vi "GetData.vi"(8 "File":path=path "10 Ft", 11 "file (use dialog)":path) -> (0 "Acceleration Limit (fps^2)":dbl, 1 "Sample Period (s)":dbl, 2 "Velocity Limit (fps)":dbl, 3 "Trajectory Data":T4(array[cluster]), 4 "Commands":cluster{"Time (s)":dbl, T2, bool}[](array[cluster]), 5 "Points":cluster{"x":dbl, "y":dbl, "th":dbl}[](array[cluster]), 6 "Description":string, 7 "Cluster":cluster{"Time (s)":dbl, "Distance (ft)":dbl}, 9 "Cluster 2":T1)   [LabVIEW 2019]
doc: "Getting trajectory data from the roboRio"
uses:
  Bordeaux/Command Stuff/Single Cmd Info.ctl
  <vilib>/picture/picture.llb/imagedata.ctl
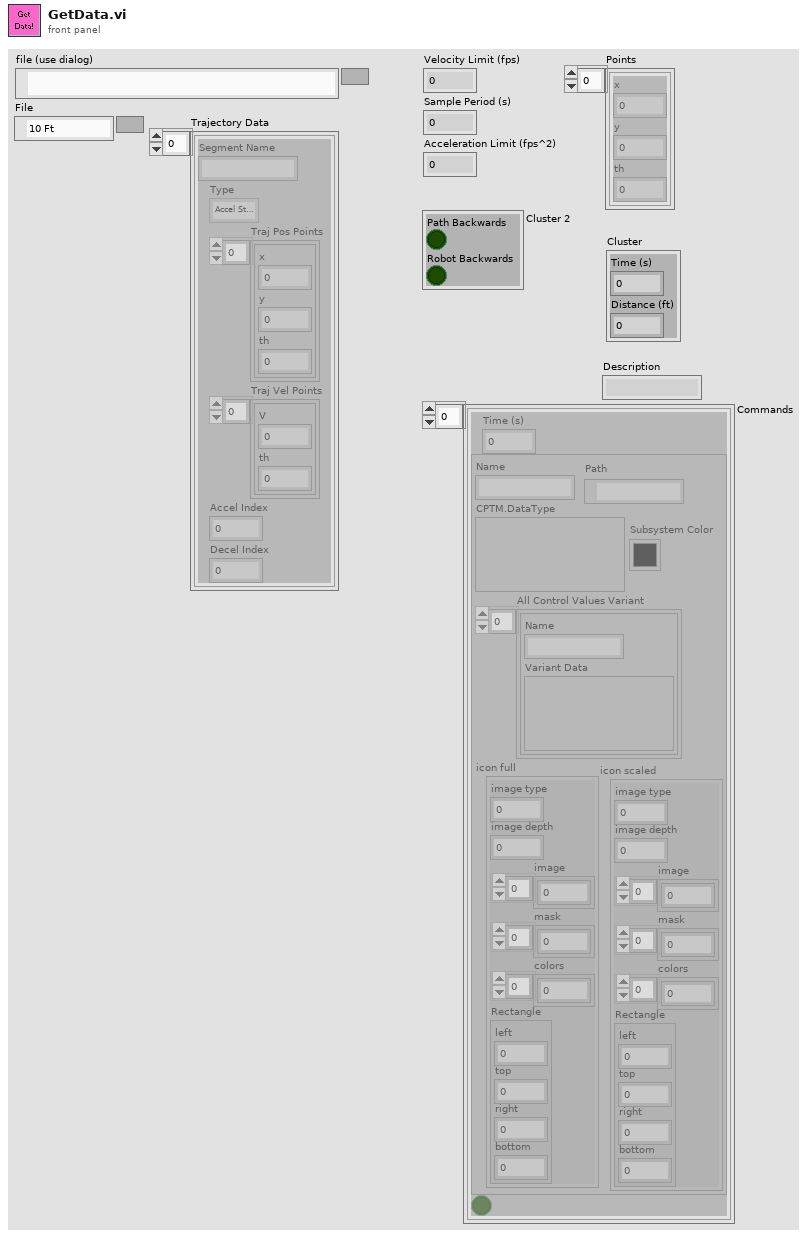
[diagram p1: front panel]
types:
  T1 = cluster{"Path Backwards":bool, "Robot Backwards":bool}
  T2 = typedef "Single Cmd Info.ctl" = cluster{"Name":string, "CPTM.DataType":variant, "All Control Values Variant":cluster{"Name":string, "Variant Data":variant}[], "icon full":T3, "icon scaled":T3, "Path":path, "Subsystem Color":u32}
  T3 = typedef "imagedata.ctl" = cluster{"image type":i32, "image depth":i32, "image":u8[], "mask":u8[], "colors":u32[], "Rectangle":cluster{"left":i16, "top":i16, "right":i16, "bottom":i16}}
  T4 = cluster{"Segment Name":string, "Type":enum16{"Accel Straight", "Const Straight", "Blend", "Circle"}, "Traj Pos Points":cluster{"x":dbl, "y":dbl, "th":dbl}[], "Traj Vel Points":cluster{"V":dbl, "th":dbl}[], "Accel Index":i32, "Decel Index":i32}[]
  T5 = cluster{"Sample Period (s)":dbl, "Limits":cluster{"Velocity (fps)":dbl, "Acceleration (fps^2)":dbl, "Jerk (fps^3)":dbl}, "Conditions":cluster{"vInitial (fps)":dbl, "vFinal (fps)":dbl}}
  T6 = cluster{"Velocity Limit (fps)":dbl, "Sample Period (s)":dbl, "Acceleration Limit (fps^2)":dbl}
  T7 = cluster{"Sample Period (s)":dbl, "Limits":cluster{"Velocity (fps)":dbl, "Acceleration (fps^2)":dbl, "Jerk (fps^3)":dbl}, "Conditions":cluster{"vInitial (fps)":dbl, "vFinal (fps)":dbl}, "Min Rads":dbl[]}
  T8 = cluster{"Sample Period (s)":dbl, "Limits":cluster{"Velocity (fps)":dbl, "Acceleration (fps^2)":dbl, "Jerk (fps^3)":dbl}, "Conditions":cluster{"vInitial (fps)":dbl, "vFinal (fps)":dbl}, "Angular Accelerations":cluster{"Angular \nAccelerations":dbl[], "Override Limits?":bool[]}}
  T9 = cluster{"Time into Path":dbl, "System":u16, "Item Selected?":bool, "System Selection":u16}[]
  T10 = cluster{"Velocity (fps)":dbl, "Acceleration (fps^2)":dbl, "Jerk (fps^3)":dbl}
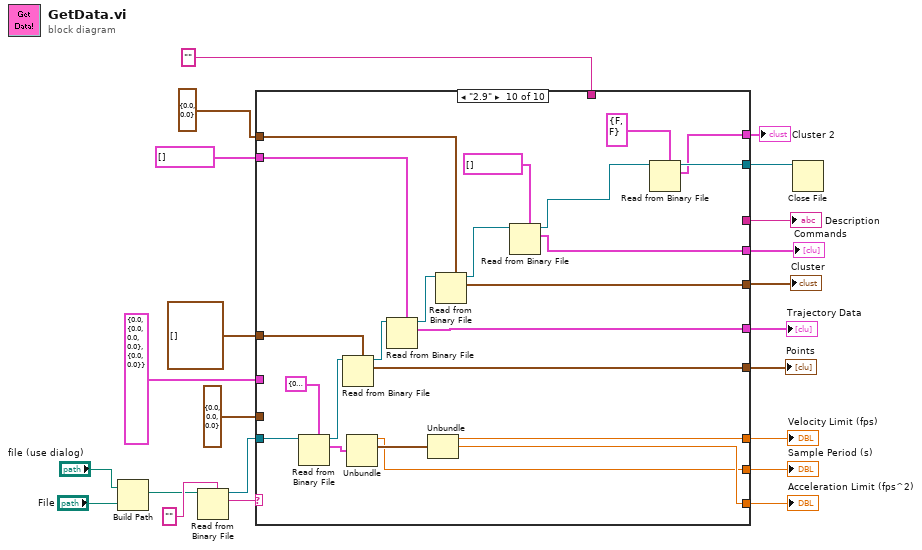
[diagram p0: block diagram]
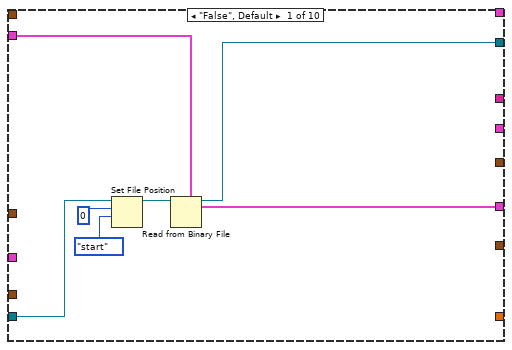
[diagram p2: hidden frame]
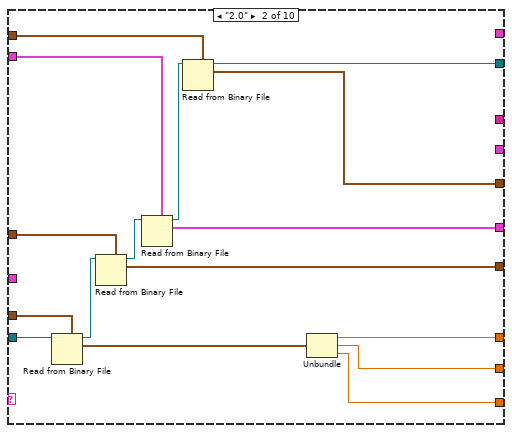
[diagram p3: hidden frame]
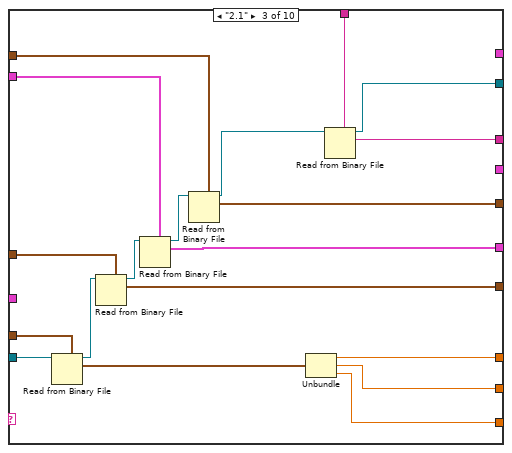
[diagram p4: hidden frame]
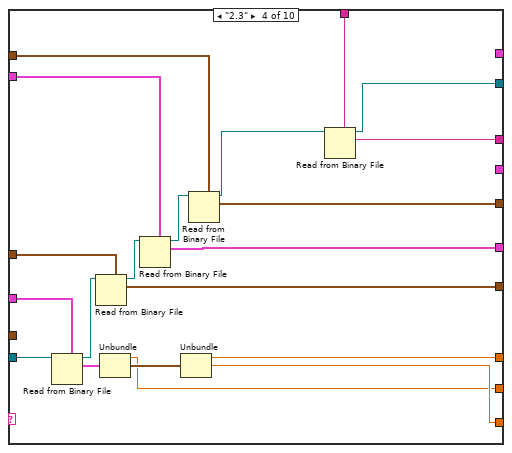
[diagram p5: hidden frame]
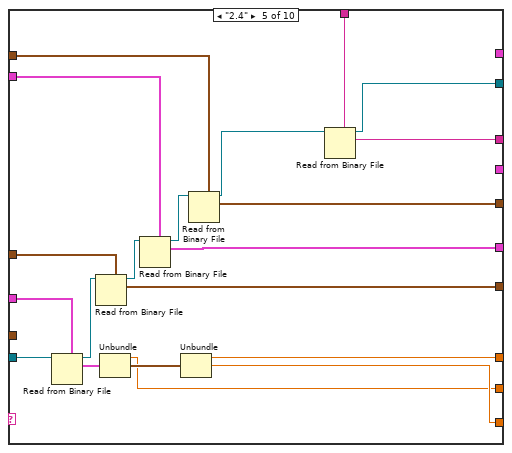
[diagram p6: hidden frame]
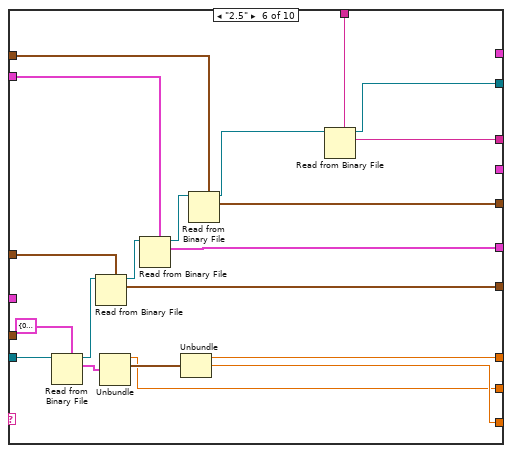
[diagram p7: hidden frame]
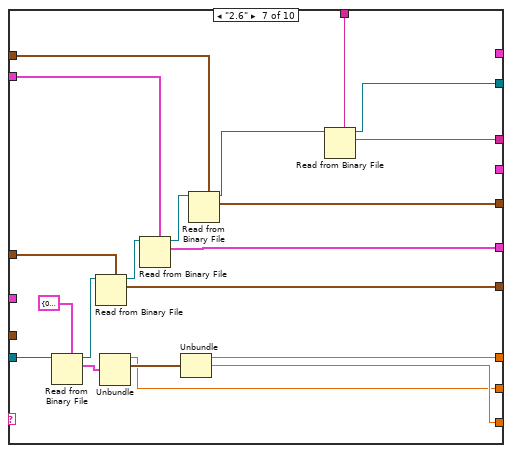
[diagram p8: hidden frame]
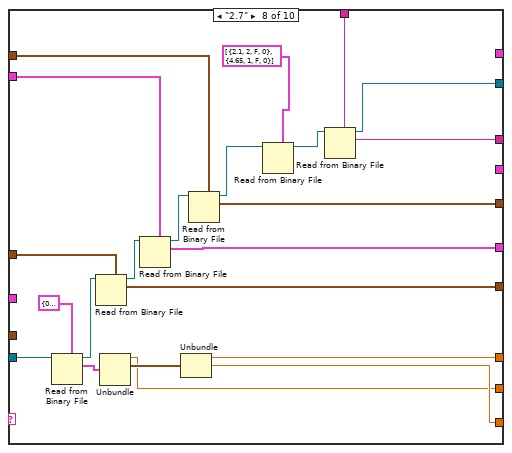
[diagram p9: hidden frame]
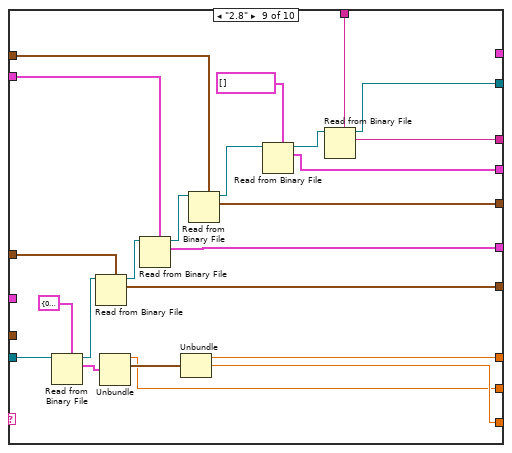
[diagram p10: hidden frame]
diagram:
  n1 = Build Path(base path="file (use dialog)", name or relative path="File") -> (appended path=w5:path)
  n2 = Read from Binary File(5:"", 11:w5) -> (2:w21:string, 3:w20:refnum<file>)  [unwired: 4 in, 2 out]
  n3 = case shown="\"2.9\"" w21 {
    tunnel: w20 -> [w24 w44 w63 w83 w103 w123 w143 w165 w188 w211]
    tunnel: T6 {"Velocity Limit (fps)"=0.0, "Sample Period (s)"=0.0, "Acceleration Limit (fps^2)"=0.0} -> [_ w43 w62 _ _ _ _ _ _ _]
    tunnel: cluster{"x":dbl, "y":dbl, "th":dbl}[] [] ("Points") -> [_ w41 w60 w81 w101 w121 w141 w163 w186 w209]
    tunnel: [_ w40 w59 w80 w100 w120 w140 w162 w185 w208] -> w11
    tunnel: T4 [] ("Trajectory Data") -> [w26 w39 w58 w79 w99 w119 w139 w161 w184 w207]
    tunnel: [w25 w37 w56 w77 w97 w117 w137 w159 w182 w205] -> w10
    tunnel: cluster{"Time (s)":dbl, "Distance (ft)":dbl} {"Time (s)"=0.0, "Distance (ft)"=0.0} -> [_ w36 w55 w76 w96 w116 w136 w158 w181 w204]
    tunnel: [_ w34 w53 w74 w94 w114 w134 w156 w179 w202] -> w9
    tunnel: [w23 w33 w48 w72 w92 w112 w132 w155 w178 w193] -> w18
    tunnel: [_ w32 w52 w67 w87 w108 w128 w151 w174 w200] -> w14
    tunnel: [_ w31 w51 w65 w85 w106 w126 w149 w172 w198] -> w13
    tunnel: [_ w30 w50 w66 w86 w107 w127 w150 w173 w199] -> w12
    tunnel: "" -> [_ _ w47 w71 w91 w111 w131 w154 w177 _]
    tunnel: [_ _ w46 w70 w90 w110 w130 w153 w176 _] -> w7
    tunnel: T5 {"Sample Period (s)"=0.0, "Limits"={"Velocity (fps)"=0.0, "Acceleration (fps^2)"=0.0, "Jerk (fps^3)"=0.0}, "Conditions"={"vInitial (fps)"=0.0, "vFinal (fps)"=0.0}} -> [_ _ _ w69 w89 _ _ _ _ _]
    tunnel: [_ _ _ _ _ _ _ _ w167 w194] -> w2
    tunnel: [_ _ _ _ _ _ _ _ _ w191] -> w1
    frame "False", Default {
      n4 = Set File Position(offset (in bytes) (0)=i64 0, refnum=w24, from (0:start)=enum16{"start", "end", "current"}."start") -> (refnum out=w27:refnum<file>)  [unwired: 1 in, 1 out]
      n5 = Read from Binary File(5:w26, 11:w27) -> (2:w25:T4, 3:w23:refnum<file>)  [unwired: 4 in, 2 out]
    }
    frame "2.0" {
      n6 = Read from Binary File(5:w43, 11:w44) -> (2:w45:T6, 3:w42:refnum<file>)  [unwired: 4 in, 2 out]
      n7 = Read from Binary File(5:w41, 11:w42) -> (2:w40:cluster{"x":dbl, "y":dbl, "th":dbl}[], 3:w38:refnum<file>)  [unwired: 4 in, 2 out]
      n8 = Read from Binary File(5:w39, 11:w38) -> (2:w37:T4, 3:w35:refnum<file>)  [unwired: 4 in, 2 out]
      n9 = Read from Binary File(5:w36, 11:w35) -> (2:w34:cluster{"Time (s)":dbl, "Distance (ft)":dbl}, 3:w33:refnum<file>)  [unwired: 4 in, 2 out]
      n10 = Unbundle(w45) -> ("Velocity Limit (fps)"=w32:dbl, "Sample Period (s)"=w31:dbl, "Acceleration Limit (fps^2)"=w30:dbl)
    }
    frame "2.1" {
      n11 = Read from Binary File(5:w62, 11:w63) -> (2:w64:T6, 3:w61:refnum<file>)  [unwired: 4 in, 2 out]
      n12 = Read from Binary File(5:w60, 11:w61) -> (2:w59:cluster{"x":dbl, "y":dbl, "th":dbl}[], 3:w57:refnum<file>)  [unwired: 4 in, 2 out]
      n13 = Read from Binary File(5:w58, 11:w57) -> (2:w56:T4, 3:w54:refnum<file>)  [unwired: 4 in, 2 out]
      n14 = Read from Binary File(5:w55, 11:w54) -> (2:w53:cluster{"Time (s)":dbl, "Distance (ft)":dbl}, 3:w49:refnum<file>)  [unwired: 4 in, 2 out]
      n15 = Unbundle(w64) -> ("Velocity Limit (fps)"=w52:dbl, "Sample Period (s)"=w51:dbl, "Acceleration Limit (fps^2)"=w50:dbl)
      n16 = Read from Binary File(5:w47, 11:w49) -> (2:w46:string, 3:w48:refnum<file>)  [unwired: 4 in, 2 out]
    }
    frame "2.3" {
      n17 = Read from Binary File(5:w69, 11:w83) -> (2:w84:T5, 3:w82:refnum<file>)  [unwired: 4 in, 2 out]
      n18 = Read from Binary File(5:w81, 11:w82) -> (2:w80:cluster{"x":dbl, "y":dbl, "th":dbl}[], 3:w78:refnum<file>)  [unwired: 4 in, 2 out]
      n19 = Unbundle(w84) -> ("Sample Period (s)"=w65:dbl, "Limits"=w68:T10)  [unwired: 1 out]
      n20 = Read from Binary File(5:w79, 11:w78) -> (2:w77:T4, 3:w75:refnum<file>)  [unwired: 4 in, 2 out]
      n21 = Unbundle(w68) -> ("Velocity (fps)"=w67:dbl, "Acceleration (fps^2)"=w66:dbl)  [unwired: 1 out]
      n22 = Read from Binary File(5:w76, 11:w75) -> (2:w74:cluster{"Time (s)":dbl, "Distance (ft)":dbl}, 3:w73:refnum<file>)  [unwired: 4 in, 2 out]
      n23 = Read from Binary File(5:w71, 11:w73) -> (2:w70:string, 3:w72:refnum<file>)  [unwired: 4 in, 2 out]
    }
    frame "2.4" {
      n24 = Read from Binary File(5:w89, 11:w103) -> (2:w104:T5, 3:w102:refnum<file>)  [unwired: 4 in, 2 out]
      n25 = Read from Binary File(5:w101, 11:w102) -> (2:w100:cluster{"x":dbl, "y":dbl, "th":dbl}[], 3:w98:refnum<file>)  [unwired: 4 in, 2 out]
      n26 = Unbundle(w104) -> ("Sample Period (s)"=w85:dbl, "Limits"=w88:T10)  [unwired: 1 out]
      n27 = Read from Binary File(5:w99, 11:w98) -> (2:w97:T4, 3:w95:refnum<file>)  [unwired: 4 in, 2 out]
      n28 = Unbundle(w88) -> ("Velocity (fps)"=w87:dbl, "Acceleration (fps^2)"=w86:dbl)  [unwired: 1 out]
      n29 = Read from Binary File(5:w96, 11:w95) -> (2:w94:cluster{"Time (s)":dbl, "Distance (ft)":dbl}, 3:w93:refnum<file>)  [unwired: 4 in, 2 out]
      n30 = Read from Binary File(5:w91, 11:w93) -> (2:w90:string, 3:w92:refnum<file>)  [unwired: 4 in, 2 out]
    }
    frame "2.5" {
      n31 = Read from Binary File(5:T7 {"Sample Period (s)"=0.0, "Limits"={"Velocity (fps)"=0.0, "Acceleration (fps^2)"=0.0, "Jerk (fps^3)"=0.0}, "Conditions"={"vInitial (fps)"=0.0, "vFinal (fps)"=0.0}, "Min Rads"=[20.0, 20.0, 20.0, 20.0, 20.0]}, 11:w123) -> (2:w124:T7, 3:w122:refnum<file>)  [unwired: 4 in, 2 out]
      n32 = Read from Binary File(5:w121, 11:w122) -> (2:w120:cluster{"x":dbl, "y":dbl, "th":dbl}[], 3:w118:refnum<file>)  [unwired: 4 in, 2 out]
      n33 = Unbundle(w124) -> ("Sample Period (s)"=w106:dbl, "Limits"=w109:T10)  [unwired: 2 out]
      n34 = Read from Binary File(5:w119, 11:w118) -> (2:w117:T4, 3:w115:refnum<file>)  [unwired: 4 in, 2 out]
      n35 = Unbundle(w109) -> ("Velocity (fps)"=w108:dbl, "Acceleration (fps^2)"=w107:dbl)  [unwired: 1 out]
      n36 = Read from Binary File(5:w116, 11:w115) -> (2:w114:cluster{"Time (s)":dbl, "Distance (ft)":dbl}, 3:w113:refnum<file>)  [unwired: 4 in, 2 out]
      n37 = Read from Binary File(5:w111, 11:w113) -> (2:w110:string, 3:w112:refnum<file>)  [unwired: 4 in, 2 out]
    }
    frame "2.6" {
      n38 = Read from Binary File(5:T8 {"Sample Period (s)"=0.0, "Limits"={"Velocity (fps)"=0.0, "Acceleration (fps^2)"=0.0, "Jerk (fps^3)"=0.0}, "Conditions"={"vInitial (fps)"=0.0, "vFinal (fps)"=0.0}, "Angular Accelerations"={"Angular \nAccelerations"=[], "Override Limits?"=[]}}, 11:w143) -> (2:w144:T8, 3:w142:refnum<file>)  [unwired: 4 in, 2 out]
      n39 = Read from Binary File(5:w141, 11:w142) -> (2:w140:cluster{"x":dbl, "y":dbl, "th":dbl}[], 3:w138:refnum<file>)  [unwired: 4 in, 2 out]
      n40 = Unbundle(w144) -> ("Sample Period (s)"=w126:dbl, "Limits"=w129:T10)  [unwired: 2 out]
      n41 = Read from Binary File(5:w139, 11:w138) -> (2:w137:T4, 3:w135:refnum<file>)  [unwired: 4 in, 2 out]
      n42 = Unbundle(w129) -> ("Velocity (fps)"=w128:dbl, "Acceleration (fps^2)"=w127:dbl)  [unwired: 1 out]
      n43 = Read from Binary File(5:w136, 11:w135) -> (2:w134:cluster{"Time (s)":dbl, "Distance (ft)":dbl}, 3:w133:refnum<file>)  [unwired: 4 in, 2 out]
      n44 = Read from Binary File(5:w131, 11:w133) -> (2:w130:string, 3:w132:refnum<file>)  [unwired: 4 in, 2 out]
    }
    frame "2.7" {
      n45 = Read from Binary File(5:T8 {"Sample Period (s)"=0.0, "Limits"={"Velocity (fps)"=0.0, "Acceleration (fps^2)"=0.0, "Jerk (fps^3)"=0.0}, "Conditions"={"vInitial (fps)"=0.0, "vFinal (fps)"=0.0}, "Angular Accelerations"={"Angular \nAccelerations"=[], "Override Limits?"=[]}}, 11:w165) -> (2:w166:T8, 3:w164:refnum<file>)  [unwired: 4 in, 2 out]
      n46 = Read from Binary File(5:w163, 11:w164) -> (2:w162:cluster{"x":dbl, "y":dbl, "th":dbl}[], 3:w160:refnum<file>)  [unwired: 4 in, 2 out]
      n47 = Unbundle(w166) -> ("Sample Period (s)"=w149:dbl, "Limits"=w152:T10)  [unwired: 2 out]
      n48 = Read from Binary File(5:w161, 11:w160) -> (2:w159:T4, 3:w157:refnum<file>)  [unwired: 4 in, 2 out]
      n49 = Unbundle(w152) -> ("Velocity (fps)"=w151:dbl, "Acceleration (fps^2)"=w150:dbl)  [unwired: 1 out]
      n50 = Read from Binary File(5:w158, 11:w157) -> (2:w156:cluster{"Time (s)":dbl, "Distance (ft)":dbl}, 3:w147:refnum<file>)  [unwired: 4 in, 2 out]
      n51 = Read from Binary File(5:T9 [{"Time into Path"=2.1, "System"=2, "Item Selected?"=FALSE, "System Selection"=0}, {"Time into Path"=4.65, "System"=1, "Item Selected?"=FALSE, "System Selection"=0}] ("Commands"), 11:w147) -> (3:w146:refnum<file>)  [unwired: 4 in, 3 out]
      n52 = Read from Binary File(5:w154, 11:w146) -> (2:w153:string, 3:w155:refnum<file>)  [unwired: 4 in, 2 out]
    }
    frame "2.8" {
      n53 = Read from Binary File(5:T8 {"Sample Period (s)"=0.0, "Limits"={"Velocity (fps)"=0.0, "Acceleration (fps^2)"=0.0, "Jerk (fps^3)"=0.0}, "Conditions"={"vInitial (fps)"=0.0, "vFinal (fps)"=0.0}, "Angular Accelerations"={"Angular \nAccelerations"=[], "Override Limits?"=[]}}, 11:w188) -> (2:w189:T8, 3:w187:refnum<file>)  [unwired: 4 in, 2 out]
      n54 = Read from Binary File(5:w186, 11:w187) -> (2:w185:cluster{"x":dbl, "y":dbl, "th":dbl}[], 3:w183:refnum<file>)  [unwired: 4 in, 2 out]
      n55 = Unbundle(w189) -> ("Sample Period (s)"=w172:dbl, "Limits"=w175:T10)  [unwired: 2 out]
      n56 = Read from Binary File(5:w184, 11:w183) -> (2:w182:T4, 3:w180:refnum<file>)  [unwired: 4 in, 2 out]
      n57 = Unbundle(w175) -> ("Velocity (fps)"=w174:dbl, "Acceleration (fps^2)"=w173:dbl)  [unwired: 1 out]
      n58 = Read from Binary File(5:w181, 11:w180) -> (2:w179:cluster{"Time (s)":dbl, "Distance (ft)":dbl}, 3:w170:refnum<file>)  [unwired: 4 in, 2 out]
      n59 = Read from Binary File(5:cluster{"Time (s)":dbl, T2, bool}[] [], 11:w170) -> (2:w167:cluster{"Time (s)":dbl, T2, bool}[], 3:w169:refnum<file>)  [unwired: 4 in, 2 out]
      n60 = Read from Binary File(5:w177, 11:w169) -> (2:w176:string, 3:w178:refnum<file>)  [unwired: 4 in, 2 out]
    }
    frame "2.9" {
      n61 = Read from Binary File(5:T8 {"Sample Period (s)"=0.0, "Limits"={"Velocity (fps)"=0.0, "Acceleration (fps^2)"=0.0, "Jerk (fps^3)"=0.0}, "Conditions"={"vInitial (fps)"=0.0, "vFinal (fps)"=0.0}, "Angular Accelerations"={"Angular \nAccelerations"=[], "Override Limits?"=[]}}, 11:w211) -> (2:w212:T8, 3:w210:refnum<file>)  [unwired: 4 in, 2 out]
      n62 = Read from Binary File(5:w209, 11:w210) -> (2:w208:cluster{"x":dbl, "y":dbl, "th":dbl}[], 3:w206:refnum<file>)  [unwired: 4 in, 2 out]
      n63 = Unbundle(w212) -> ("Sample Period (s)"=w198:dbl, "Limits"=w201:T10)  [unwired: 2 out]
      n64 = Read from Binary File(5:w207, 11:w206) -> (2:w205:T4, 3:w203:refnum<file>)  [unwired: 4 in, 2 out]
      n65 = Unbundle(w201) -> ("Velocity (fps)"=w200:dbl, "Acceleration (fps^2)"=w199:dbl)  [unwired: 1 out]
      n66 = Read from Binary File(5:w204, 11:w203) -> (2:w202:cluster{"Time (s)":dbl, "Distance (ft)":dbl}, 3:w196:refnum<file>)  [unwired: 4 in, 2 out]
      n67 = Read from Binary File(5:cluster{"Time (s)":dbl, T2, bool}[] [], 11:w196) -> (2:w194:cluster{"Time (s)":dbl, T2, bool}[], 3:w190:refnum<file>)  [unwired: 4 in, 2 out]
      n68 = Read from Binary File(5:T1 {"Path Backwards"=FALSE, "Robot Backwards"=FALSE} ("Cluster"), 11:w190) -> (2:w191:T1, 3:w193:refnum<file>)  [unwired: 4 in, 2 out]
    }
  }
  "Velocity Limit (fps)" <- w14
  "Sample Period (s)" <- w13
  "Acceleration Limit (fps^2)" <- w12
  "Points" <- w11
  "Trajectory Data" <- w10
  "Cluster" <- w9
  "Description" <- w7
  "Commands" <- w2
  "Cluster 2" <- w1
  n69 = Close File(refnum=w18) -> ()  [unwired: 1 in, 2 out]
